vi "SaveWaveforms.vi"(0 "LXe Level":dbl, 1 "Save File":path, 2 "Array":refnum<vi>[](array[refnum]), 3 "Time Stamp":timestamp) -> ()   [LabVIEW 2023]
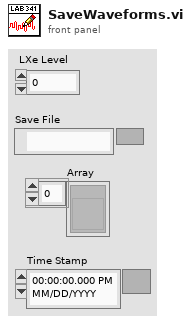
[diagram p1: front panel]
types:
  T1 = cluster{"Time Stamp":timestamp, "History Data":dbl[][], "LXe Level":dbl}
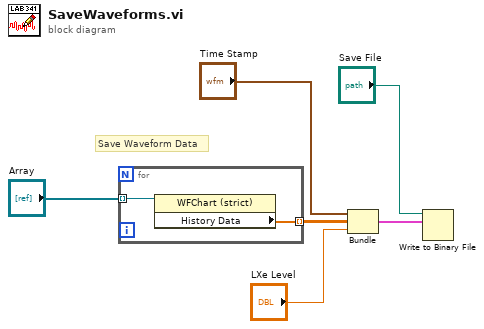
[diagram p0: block diagram]
diagram:
  # "Save Waveform Data"
  n1 = for {
    tunnel: "Array" -> [w8] mode=indexing
    tunnel: [w7] -> w6 mode=indexing
    n2 = property on="Property Node" class="WFChart (strict)"(reference=w8) -> ("History Data"=w7:dbl[])  [unwired: 1 in, 2 out]
  }
  n3 = Bundle("Time Stamp"="Time Stamp", "History Data"=w6, "LXe Level"="LXe Level") -> (w5:T1)  [unwired: 1 in]
  n4 = Write to Binary File(file (use dialog)="Save File", data=w5) -> ()  [unwired: 4 in, 3 out]
